vi "Shift Register 0 dan 4 e kadar sayılar toplamı programı for - while döngüsü.vi"() -> ()   [LabVIEW 2014]
panel:
  out "Numeric 2":dbl
  out "Numeric":dbl
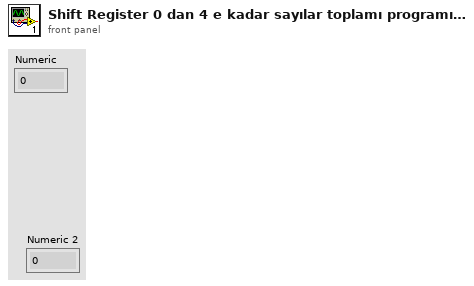
[diagram p1: front panel]
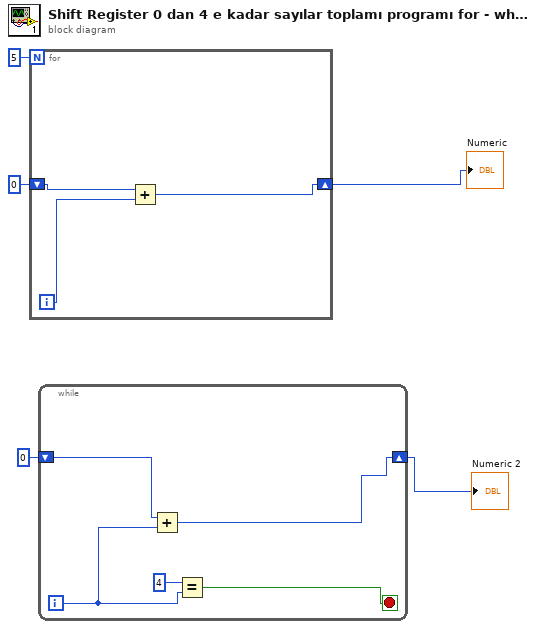
[diagram p0: block diagram]
diagram:
  n1 = for {
    N: 5 -> [_]
    shift-right: [w7] -> w4
    shift-left: 0 -> [w6]
    i -> [w8]
    n2 = Add(x=w6, y=w8) -> (x+y=w7:i32)
  }
  "Numeric" <- w4
  n3 = while {
    shift-right: [w13] -> w1
    shift-left: 0 -> [w12]
    i -> [w9]
    stop <- w11 stop-if-true
    n4 = Add(x=w12, y=w9) -> (x+y=w13:i32)
    n5 = Equal?(x=4, y=w9) -> (x = y?=w11:bool)
  }
  "Numeric 2" <- w1
